vi "CMD_Drive.vi"(1 "Line":string) -> (0 "Done":bool)   [LabVIEW 2015]
uses:
  <vilib>/Rock Robotics/WPI/Utilities/WPI_GetSetVariantRefNum.vi
  <vilib>/Rock Robotics/Network Tables/NT Read Number.vi
panel:
  out "error":string
  in  "Parameters":i32[](array[numeric])=[1, 2, 1, 1, 0, 1]
  in  "Subcommands":string[](array[string])=["for", "at", "until", "to", "align", "turn"]
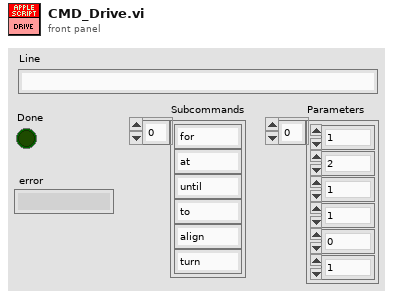
[diagram p1: front panel]
types:
  T1 = typedef "WPI_RobotDriveDevRef.ctl" = cluster{"DevStatus":errorcluster, "Motors[]":T2[], "Square Inputs":bool, "Max Output":dbl}
  T2 = typedef "WPI_MotorControlDeviceRef.ctl" = cluster{"DeviceStatus":errorcluster, "Type":T3, "PWM":cluster{"PWM Channel":T4, "DeadBand":T5}, "CAN":cluster{"Device Number":u8, "Control Mode":T6, "Semaphore":T7, "Max Vout":dbl, "TalonSRX Control Mode":T8}, "Invert":bool}
  T3 = typedef "WPI_MotorControlType.ctl" = enum16{"PWM", "CAN", "CANTalonSRX"}
  T4 = typedef "FPGA_DIOPWMChannel.ctl" = enum8{"PWM 0", "PWM 1", "PWM 2", "PWM 3", "PWM 4", "PWM 5", "PWM 6", "PWM 7", "PWM 8", "PWM 9", "PWM MXP 0", "PWM MXP 1", "PWM MXP 2", "PWM MXP 3", "PWM MXP 4", "PWM MXP 5", "PWM MXP 6", "PWM MXP 7", "PWM MXP 8", "PWM MXP 9", "Invalid"}
  T5 = typedef "WPI_PWMDeadband.ctl" = cluster{"Name":string, "maxPositivePwm":i32, "minPositivePwm":i32, "centerPwm":i32, "maxNegativePwm":i32, "minNegativePwm":i32, "angularRange":u16}
  T6 = typedef "WPI_CANJaguar_ControlMode.ctl" = enum8{"Percent VBus", "Current", "Speed", "Position", "Voltage"}
  T7 = typedef "Semaphore RefNum" = refnum<k1>
  T8 = typedef "WPI_CANTalonSRX_APIControlMode.ctl" = enum8{"Percent VBus", "Speed", "Position", "Slave", "Unchanged / Invalid", "Voltage Compensation", "Current", "Motion Profile"}
  T9 = typedef "WPI_EncoderDevRef.ctl" = cluster{"DevStatus":errorcluster, "EncoderIndex":T10, "CounterIndex":T11, "DistancePerCount":dbl, "Decoding Type":T12}
  T10 = typedef "FPGA_EncoderIdx.ctl" = enum8{"Enc 0", "Enc 1", "Enc 2", "Enc 3", "Enc 4", "Enc 5", "Enc 6", "Enc 7", "Invalid"}
  T11 = typedef "FPGA_CounterCtrSystemIndex.ctl" = enum8{"Ctr 0", "Ctr 1", "Ctr 2", "Ctr 3", "Ctr 4", "Ctr 5", "Ctr 6", "Ctr 7", "Invalid"}
  T12 = typedef "WPI_EncoderType.ctl" = enum16{"1x", "2x", "4x"}
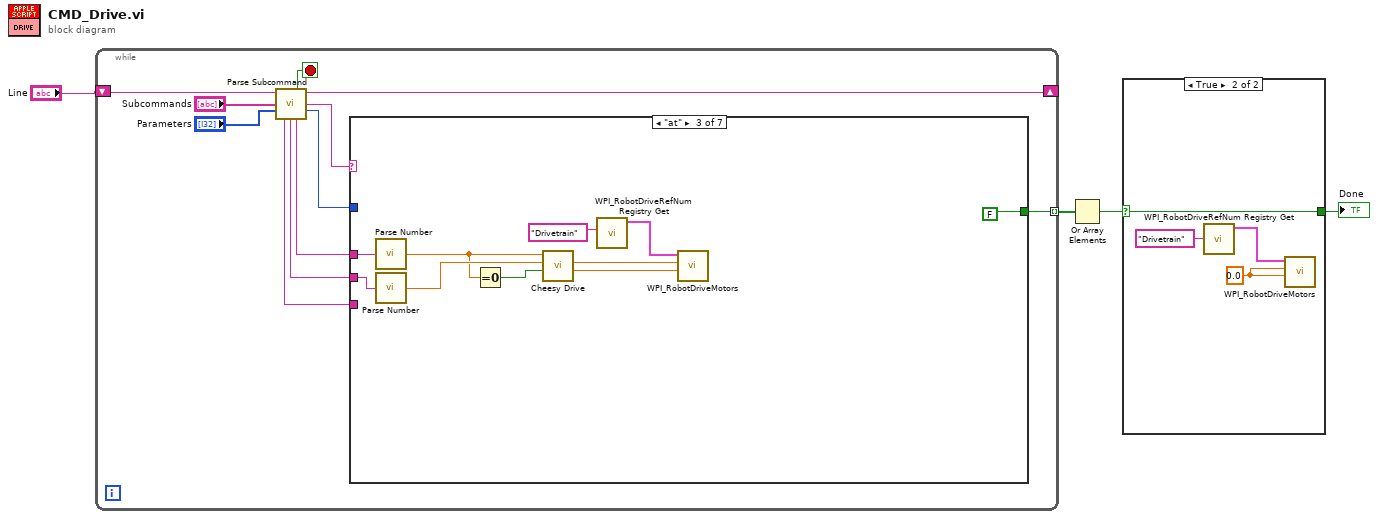
[diagram p0: block diagram]
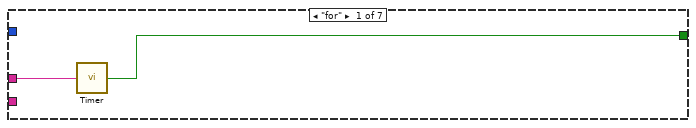
[diagram p2: hidden frame]
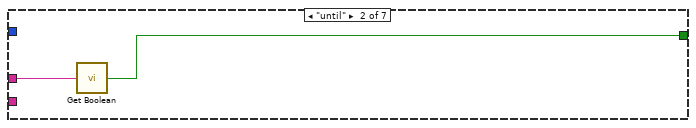
[diagram p3: hidden frame]
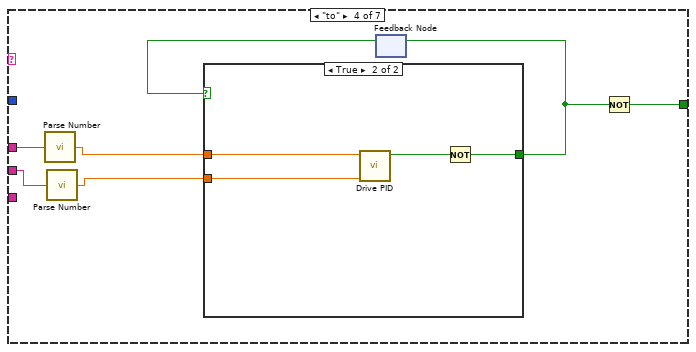
[diagram p4: hidden frame]
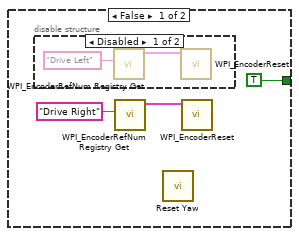
[diagram p5: hidden frame]
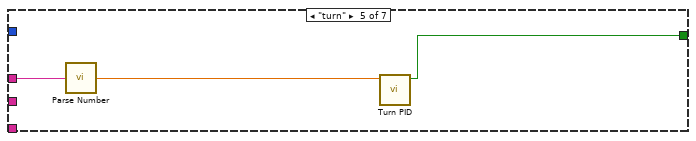
[diagram p7: hidden frame]
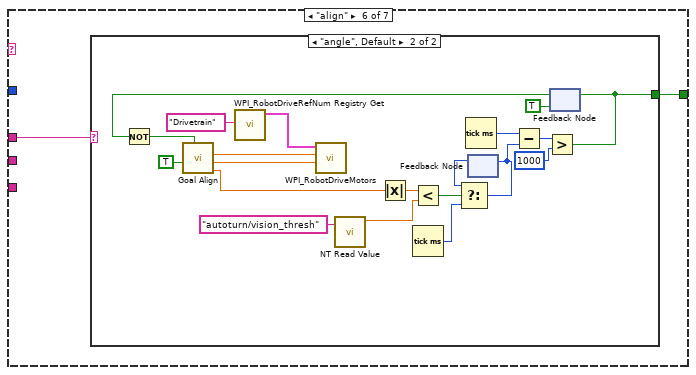
[diagram p8: hidden frame]
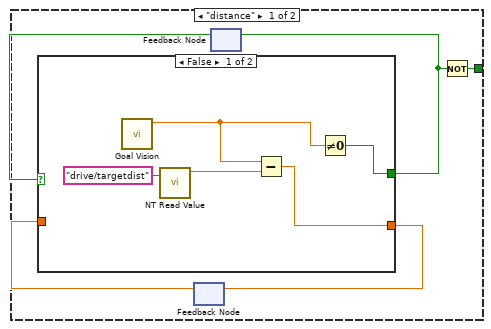
[diagram p9: hidden frame]
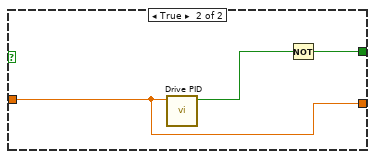
[diagram p10: hidden frame]
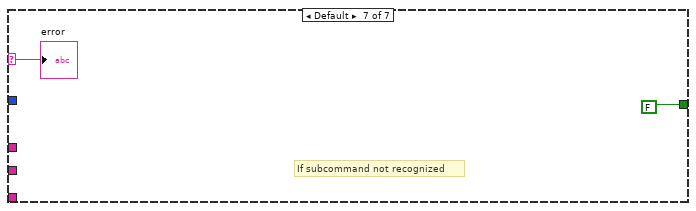
[diagram p11: hidden frame]
diagram:
  n1 = while {
    tunnel: [w15] -> w4 mode=indexing
    shift-right: [w7] -> _
    shift-left: "Line" -> [w6]
    stop <- w5 stop-if-true
    n2 = call "Parse Subcommand.vi"("Text In"=w6, "Subcommands"="Subcommands", "Parameters"="Parameters") -> ("Done"=w5:bool, "Text Out"=w7:string, "Subcommand"=w12:string, "# of Parameters"=w11:i32, "Parameter 3"=w8:string, "Parameter 2"=w9:string, "Parameter 1"=w10:string)  [unwired: 6 in]
    n3 = case shown="\"at\"" w12 {
      selector: w12 -> [_ _ _ _ _ _ w84]
      tunnel: w11 -> [_ _ _ _ _ _ _]
      tunnel: w10 -> [w17 w19 w29 w36 w48 w50 _]
      tunnel: w9 -> [_ _ w28 w31 _ _ _]
      tunnel: w8 -> [_ _ _ _ _ _ _]
      tunnel: [w16 w18 FALSE ("Value") w34 w46 w49 FALSE] -> w15
      frame "for" {
        n4 = call "Timer.vi"("Seconds (string)"=w17) -> ("Done"=w16:bool)
      }
      frame "until" {
        n5 = call "Get Boolean.vi"("Name"=w19) -> ("Value"=w18:bool)
      }
      frame "at" {
        n6 = call "Parse Number.vi"("String"=w29) -> ("Number"=w21:dbl)
        n7 = call "Parse Number.vi"("String"=w28) -> ("Number"=w27:dbl)
        n8 = Equal To 0?(x=w21) -> (x = 0?=w20:bool)
        n9 = call "Cheesy Drive.vi"("Quickturn"=w20, "Turn"=w27, "Throttle"=w21) -> ("Right"=w24:dbl, "Left"=w25:dbl)  [unwired: 5 in]
        n10 = call <vilib>:"WPI_RobotDriveRefNum Registry Get.vi"("refnum name"="Drivetrain") -> ("RobotDriveDevRef"=w26:T1)  [unwired: 9 in, 1 out]
        n11 = call <vilib>:"WPI_RobotDriveMotors.vi"("RightSpeed"=w24, "LeftSpeed"=w25, "RobotDriveDevRef"=w26) -> ()  [unwired: 6 in, 3 out]
      }
      frame "to" {
        n12 = call "Parse Number.vi"("String"=w36) -> ("Number"=w33:dbl)
        n13 = call "Parse Number.vi"("String"=w31) -> ("Number"=w30:dbl)
        n14 = feedback #1() -> (w35:bool)  [unwired: 1 in]
        n15 = case shown="True" w35 {
          tunnel: [TRUE w44] -> w32
          tunnel: w33 -> [_ w43]
          tunnel: w30 -> [_ w42]
          frame False {
            n16 = disable-structure shown="Disabled" {
              frame Disabled {
                n17 = call <vilib>:"WPI_EncoderRefNum Registry Get.vi"("refnum name"="Drive Left") -> ("EncoderDevRef"=w41:T9)  [unwired: 9 in, 1 out]
                n18 = call <vilib>:"WPI_EncoderReset.vi"("EncoderDevRef"=w41) -> ()  [unwired: 9 in, 2 out]
              }
              frame Enabled {
              }
            }
            n19 = call <vilib>:"WPI_EncoderRefNum Registry Get.vi"("refnum name"="Drive Right") -> ("EncoderDevRef"=w38:T9)  [unwired: 9 in, 1 out]
            n20 = call "Reset Yaw.vi"() -> ()  [unwired: 12 in]
            n21 = call <vilib>:"WPI_EncoderReset.vi"("EncoderDevRef"=w38) -> ()  [unwired: 9 in, 2 out]
          }
          frame True {
            n22 = call "Drive PID.vi"("Speed"=w42, "Setpoint"=w43) -> ("Done"=w45:bool)  [unwired: 9 in]
            n23 = Not(x=w45) -> (.not. x?=w44:bool)
          }
        }
        n24 = feedback-in #1(w32) -> ()
        n25 = Not(x=w32) -> (.not. x?=w34:bool)
      }
      frame "turn" {
        n26 = call "Parse Number.vi"("String"=w48) -> ("Number"=w47:dbl)
        n27 = call "Turn PID.vi"("Setpoint"=w47) -> ("Done"=w46:bool)  [unwired: 10 in]
      }
      frame "align" {
        n28 = case shown="\"angle\", Default" w50 {
          tunnel: [w52 w66] -> w49
          frame "distance" {
            n29 = feedback #2() -> (w55:dbl)  [unwired: 1 in]
            n30 = feedback #3() -> (w54:bool)  [unwired: 1 in]
            n31 = case shown="False" w54 {
              tunnel: w55 -> [_ w61]
              tunnel: [w56 w62] -> w51
              tunnel: [w58 w61] -> w53
              frame False {
                n32 = call "Goal Vision.vi"() -> ("Distance (in)"=w57:dbl)  [unwired: 8 in, 2 out]
                n33 = call-poly <vilib>:"NT Read Value.vi"("Name"="drive/targetdist") -> ("Numeric"=w59:dbl)  [unwired: 9 in, 1 out]
                n34 = Subtract(x=w57, y=w59) -> (x-y=w58:dbl)
                n35 = Not Equal To 0?(x=w57) -> (x != 0?=w56:bool)
              }
              frame True {
                n36 = call "Drive PID.vi"("Setpoint"=w61) -> ("Done"=w63:bool)  [unwired: 10 in]
                n37 = Not(x=w63) -> (.not. x?=w62:bool)
              }
            }
            n38 = feedback-in #2(w53) -> ()
            n39 = feedback-in #3(w51) -> ()
            n40 = Not(x=w51) -> (.not. x?=w52:bool)
          }
          frame "angle", Default {
            n41 = call <vilib>:"WPI_RobotDriveRefNum Registry Get.vi"("refnum name"="Drivetrain") -> ("RobotDriveDevRef"=w83:T1)  [unwired: 9 in, 1 out]
            n42 = call-poly <vilib>:"NT Read Value.vi"("Name"="autoturn/vision_thresh") -> ("Numeric"=w71:dbl)  [unwired: 9 in, 1 out]
            n43 = Tick Count (ms)() -> (millisecond timer value=w74:u32)
            n44 = Tick Count (ms)() -> (millisecond timer value=w76:u32)
            n45 = feedback #4() -> (w75:u32)  [unwired: 1 in]
            n46 = feedback #5(TRUE) -> (w67:bool)
            n47 = Not(x=w67) -> (.not. x?=w65:bool)
            n48 = call "Goal Align.vi"("override shooter"=TRUE, "last"=w65) -> ("Left"=w82:dbl, "Right"=w81:dbl, "turn err"=w69:dbl)  [unwired: 6 in]
            n49 = call <vilib>:"WPI_RobotDriveMotors.vi"("RightSpeed"=w81, "LeftSpeed"=w82, "RobotDriveDevRef"=w83) -> ()  [unwired: 6 in, 3 out]
            n50 = Absolute Value(x=w69) -> (abs(x)=w70:dbl)
            n51 = Less?(x=w70, y=w71) -> (x < y?=w73:bool)
            n52 = Select(t=w75, s=w73, f=w74) -> (s? t:f=w77:u32)
            n53 = feedback-in #4(w77) -> ()
            n54 = Subtract(x=w76, y=w77) -> (x-y=w78:u32)
            n55 = Greater?(x=w78, y=u32 1000) -> (0:w66:bool)
            n56 = feedback-in #5(w66) -> ()
          }
        }
      }
      frame Default {
        # "If subcommand not recognized"
        "error" <- w84
      }
    }
  }
  n57 = Or Array Elements(Boolean array=w4) -> (logical OR=w3:bool)
  n58 = case shown="True" w3 {
    selector: w3 -> [w86 w88]
    tunnel: [w86 w88] -> w2
    frame False {
    }
    frame True {
      w89 = 0.0
      n59 = call <vilib>:"WPI_RobotDriveRefNum Registry Get.vi"("refnum name"="Drivetrain") -> ("RobotDriveDevRef"=w90:T1)  [unwired: 9 in, 1 out]
      n60 = call <vilib>:"WPI_RobotDriveMotors.vi"("RightSpeed"=w89, "LeftSpeed"=w89, "RobotDriveDevRef"=w90) -> ()  [unwired: 6 in, 3 out]
    }
  }
  "Done" <- w2
